vi "CoordinateTransform_InvertMatrix.vi"(2 "error in (no error)":errorcluster, 3 "Conversion Matrix":dbl[][](array[numeric])) -> (0 "error out":errorcluster, 1 "invers Conversion Matrix":dbl[][](array[numeric]))   [LabVIEW 2011]
uses:
  <vilib>/Analysis/baseanly.llb/Real Inverse Matrix.vi
  <vilib>/Analysis/NI_AALBase.lvlib
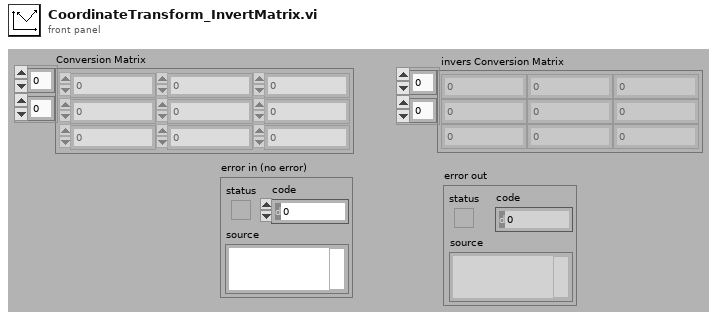
[diagram p1: front panel]
types:
  T1 = typedef "NI_Matrix.lvlib/RealMatrix.ctl" = dbl[][]
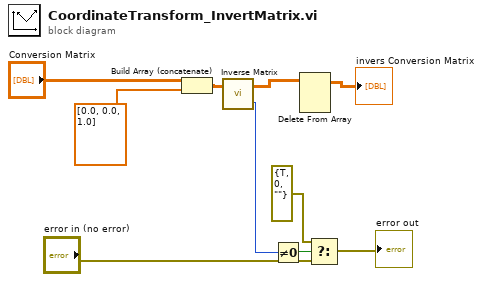
[diagram p0: block diagram]
diagram:
  n1 = Build Array (concatenate)("Conversion Matrix", dbl[] [0.0, 0.0, 1.0]) -> (w9:dbl[][])
  n2 = call-poly <vilib>:"Inverse Matrix.vi"("Input Matrix"=w9) -> ("error"=w6:i32, "Inverse Matrix"=w1:T1)  [unwired: 1 in]
  n3 = Not Equal To 0?(x=w6) -> (x != 0?=w7:bool)
  n4 = Delete From Array(array=w1) -> (array with subset deleted=→"invers Conversion Matrix":T1)  [unwired: 3 in, 1 out]
  n5 = Select(t=errorcluster {"status"=TRUE, "code"=0, "source"=""}, s=w7, f="error in (no error)") -> (s? t:f=→"error out":errorcluster)
